vi "HW5p1_Task1_nguyejk.vi"() -> ()   [LabVIEW 2016]
panel:
  in  "b":dbl
  in  "a":dbl
  in  "Pv":dbl
  out "D":dbl
  in  "r":dbl
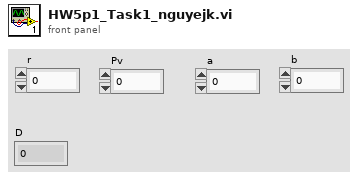
[diagram p1: front panel]
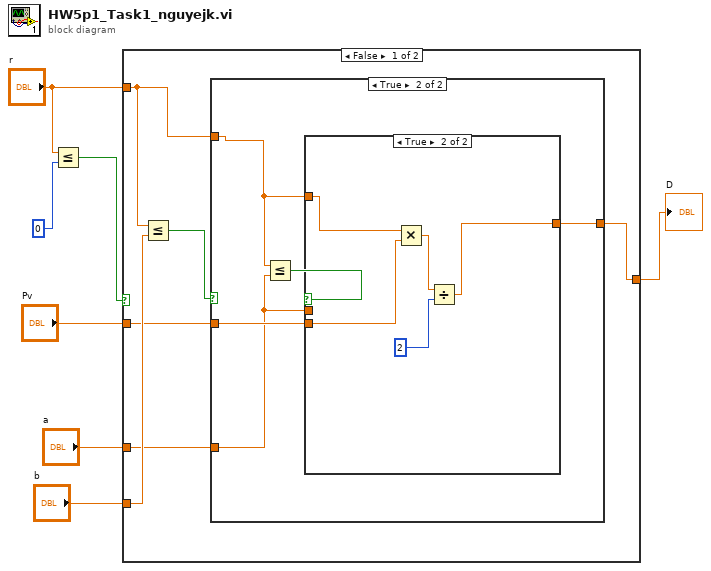
[diagram p0: block diagram]
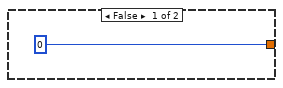
[diagram p2: hidden frame]
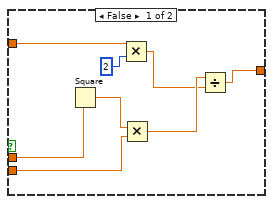
[diagram p3: hidden frame]
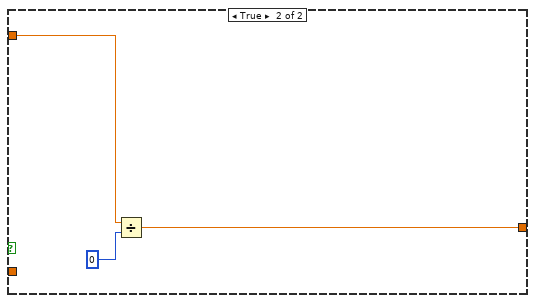
[diagram p4: hidden frame]
diagram:
  n1 = Less Or Equal?(x="r", y=0) -> (x <= y?=w6:bool)
  n2 = case shown="False" w6 {
    tunnel: "r" -> [w11 w35]
    tunnel: [w12 w33] -> w4
    tunnel: "b" -> [w10 _]
    tunnel: "a" -> [w9 _]
    tunnel: "Pv" -> [w8 _]
    frame False {
      n3 = Less Or Equal?(x=w11, y=w10) -> (x <= y?=w13:bool)
      n4 = case shown="True" w13 {
        tunnel: [0 w17] -> w12
        tunnel: w11 -> [_ w15]
        tunnel: w9 -> [_ w16]
        tunnel: w8 -> [_ w18]
        frame False {
        }
        frame True {
          n5 = Less Or Equal?(x=w15, y=w16) -> (x <= y?=w19:bool)
          n6 = case shown="True" w19 {
            tunnel: w15 -> [w25 w28]
            tunnel: w18 -> [w23 w31]
            tunnel: [w20 w29] -> w17
            tunnel: w16 -> [w27 _]
            frame False {
              n7 = Square(x=w27) -> (x^2=w26:dbl)
              n8 = Multiply(x=w25, y=2) -> (x*y=w21:dbl)
              n9 = Multiply(x=w26, y=w23) -> (x*y=w22:dbl)
              n10 = Divide(x=w22, y=w21) -> (x/y=w20:dbl)
            }
            frame True {
              n11 = Multiply(x=w28, y=w31) -> (x*y=w30:dbl)
              n12 = Divide(x=w30, y=2) -> (x/y=w29:dbl)
            }
          }
        }
      }
    }
    frame True {
      n13 = Divide(x=w35, y=0) -> (x/y=w33:dbl)
    }
  }
  "D" <- w4
